vi "闹钟（多分）.vi"(5 "设置分":i32[](array[numeric]), 7 "启用":bool=TRUE) -> (6 "时间到脉冲":bool, 8 "分":i32)   [LabVIEW 2012]
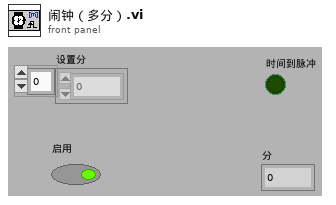
[diagram p1: front panel]
types:
  T1 = typedef "LVDateTimeRec.ctl" = cluster{"秒数的小数部分":dbl, "秒":i32, "分":i32, "时":i32, "日":i32, "月":i32, "年":i32, "天数（周）":i32, "天数（年）":i32, "DST":i32}
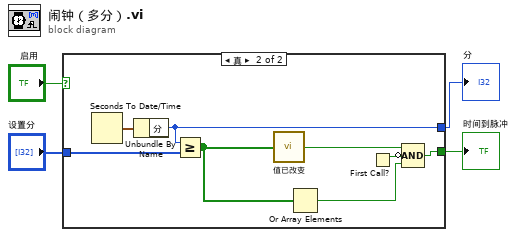
[diagram p0: block diagram]
diagram:
  n1 = case shown="真" "启用" {
    tunnel: "设置分" -> [_ w9]
    tunnel: [_ w11] -> w2
    tunnel: [_ w8] -> w1
    frame False {
    }
    frame True {
      n2 = Seconds To Date/Time() -> (date time rec=w12:T1)  [unwired: 2 in]
      n3 = Unbundle By Name(w12) -> ("分"=w8:i32)
      n4 = Greater Or Equal?(x=w8, y=w9) -> (x >= y?=w6:bool[])
      n5 = call-poly "值已改变.vi"("输入数据"=w6) -> ("已更改"=w7:bool)  [unwired: 3 in]
      n6 = Or Array Elements(Boolean array=w6) -> (logical OR=w5:bool)
      n7 = First Call?() -> (First Call?: T/F=w10:bool)
      n8 = Compound Arithmetic op=AND(w7, invert w10, w5) -> (w11:bool)
    }
  }
  "时间到脉冲" <- w2
  "分" <- w1
